vi "Get HSE module.vi"(8 "error in (no error)":errorcluster, 11 "Library in":refnum<class "Library.lvclass">) -> (0 "error out":errorcluster, 2 "HSE module":bool, 3 "Library out":refnum<class "Library.lvclass">)   [LabVIEW 2020, in "Panther Dashboard.lvlib" / "Library.lvclass"]
uses:
  Library.lvclass
  Library.lvclass/Library.ctl
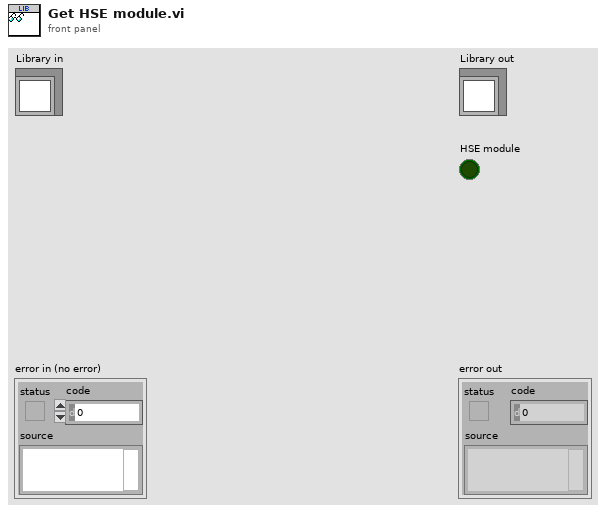
[diagram p1: front panel]
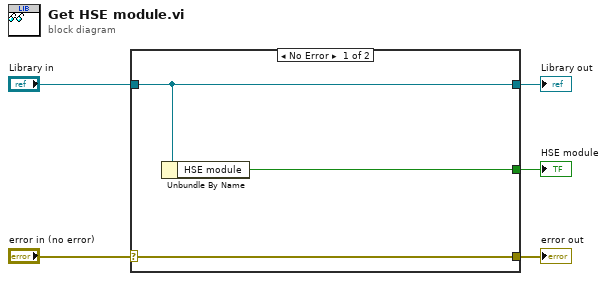
[diagram p0: block diagram]
diagram:
  n1 = case shown="No Error" "error in (no error)" {
    selector: "error in (no error)" -> [w8 w9]
    tunnel: [w8 w9] -> w4
    tunnel: [w7 w10] -> w2
    tunnel: "Library in" -> [w7 w10]
    tunnel: [w6 _] -> w1
    frame No Error {
      n2 = Unbundle By Name(w7) -> ("HSE module"=w6:bool)
    }
    frame Error {
    }
  }
  "error out" <- w4
  "Library out" <- w2
  "HSE module" <- w1
